vi "BBoxOneLabViewTest.vi"() -> ()   [LabVIEW 2019]
uses:
  Y:/Codebase/bbox-api/example/LabView2015/BBoxAPI.dll
  BBoxAPI.dll
panel:
  out "AAKit Name":string="TMYTEK_4x4"
  out "SN":string
  out "SN & IP":string[](array[string])
  out "setBeamXY":string
  in  "Ang Y":dbl
  in  "Ang X":dbl
  out "init  result":string
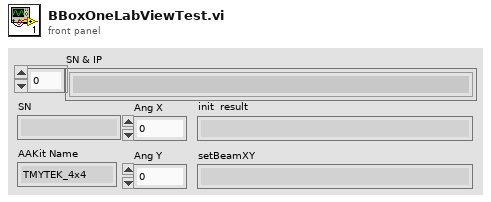
[diagram p1: front panel]
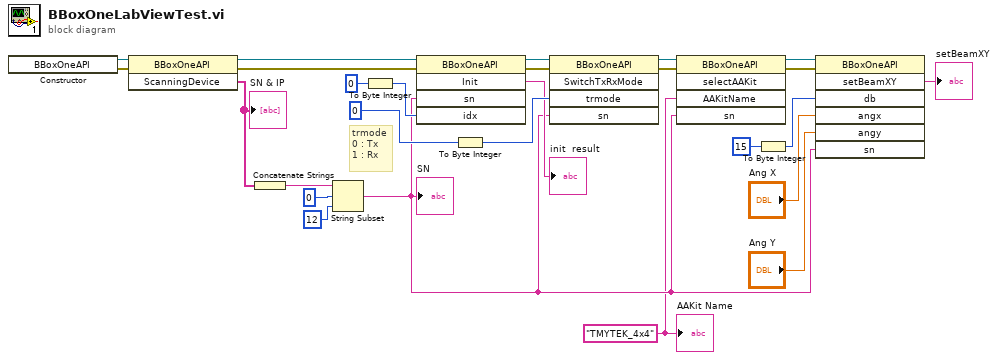
[diagram p0: block diagram]
diagram:
  w1 = "TMYTEK_4x4"
  # "trmode\n0 : Tx\n1 : Rx"
  n1 = constructor class="BBoxOneAPI"() -> (reference out=w18:refnum<k24>, error out=w17:errorcluster)  [unwired: 3 in, 1 out]
  n2 = invoke class="BBoxOneAPI" method="ScanningDevice"(reference=w18, error in=w17) -> (reference out=w16:refnum<k24>, error out=w15:errorcluster, "ScanningDevice"=w9:string[])  [unwired: 1 in]
  "SN & IP" <- w9
  n3 = Concatenate Strings(w9) -> (w8:string)
  n4 = String Subset(string=w8, offset (0)=0, length (rest)=12) -> (substring=w7:string)
  "SN" <- w7
  n5 = To Byte Integer(number=0) -> (8bit integer=w12:i8)
  n6 = invoke class="BBoxOneAPI" method="Init"(reference=w16, error in=w15, "sn"=w7, "idx"=w12) -> (reference out=w25:refnum<k24>, error out=w24:errorcluster, "Init"=→"init  result":string)  [unwired: 1 in, 2 out]
  n7 = To Byte Integer(number=0) -> (8bit integer=w22:i8)
  n8 = invoke class="BBoxOneAPI" method="SwitchTxRxMode"(reference=w25, error in=w24, "trmode"=w22, "sn"=w7) -> (reference out=w21:refnum<k24>, error out=w20:errorcluster)  [unwired: 1 in, 3 out]
  n9 = invoke class="BBoxOneAPI" method="selectAAKit"(reference=w21, error in=w20, "AAKitName"=w1, "sn"=w7) -> (reference out=w14:refnum<k24>, error out=w13:errorcluster)  [unwired: 1 in, 3 out]
  n10 = To Byte Integer(number=15) -> (8bit integer=w5:i8)
  n11 = invoke class="BBoxOneAPI" method="setBeamXY"(reference=w14, error in=w13, "db"=w5, "angx"="Ang X", "angy"="Ang Y", "sn"=w7) -> ("setBeamXY"=→"setBeamXY":string)  [unwired: 1 in, 6 out]
  "AAKit Name" <- w1
